vi "prediction_puissance.vi"() -> ()   [LabVIEW 2019]
uses:
  <vilib>/Utility/file.llb/Read Delimited Spreadsheet (DBL).vi
  <vilib>/Analysis/NI_AALPro.lvlib
panel:
  in  "Dossier ratio longueur d'ondes":path
  out "longueur d'onde":dbl
  out "XY Graph":cluster{"Y":dbl[], "Y":dbl[]}[](graph)
  in  "Dossier de tension":path
  # "on peut le remplacer par une constante dans le code"
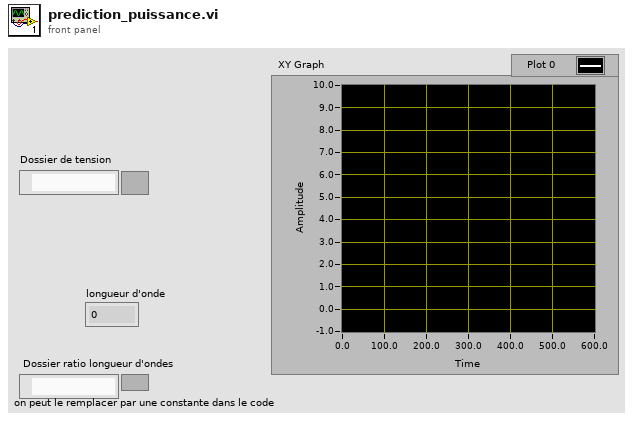
[diagram p1: front panel]
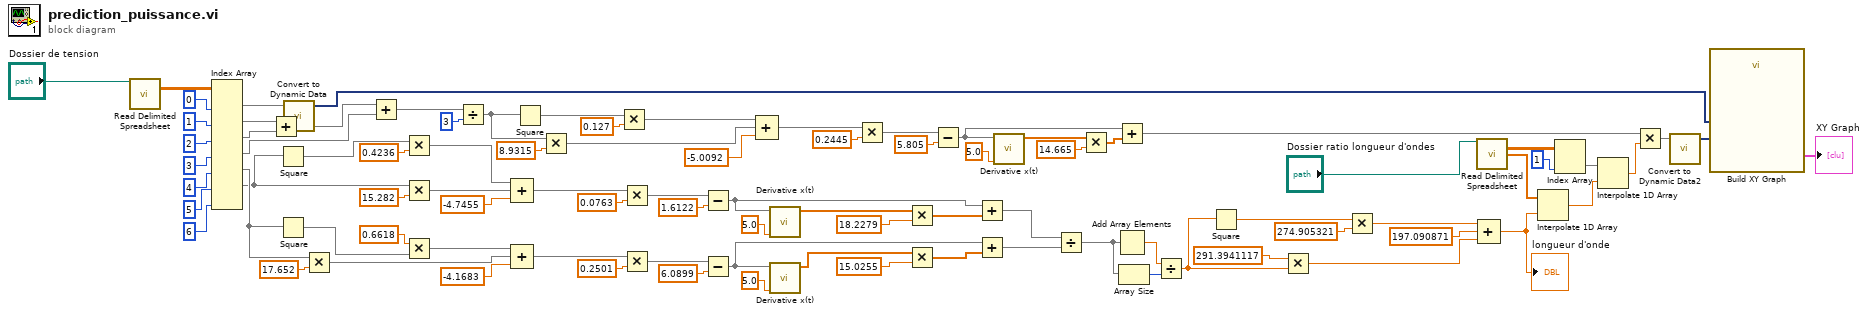
[diagram p0: block diagram]
diagram:
  n1 = call-poly <vilib>:"Read Delimited Spreadsheet.vi"("file path (dialog if empty)"="Dossier de tension") -> ("all rows"=w88:dbl[][])  [unwired: 9 in, 5 out]
  n2 = Index Array(array=w88, index (col) #1=0 ("disabled index (col)"), index (col) #2=1 ("index (col)"), index (col) #3=2 ("index (col)"), index (col) #4=3 ("index (col)"), index (col) #5=4 ("index (col)"), index (col) #6=5 ("index (col)"), index (col) #7=6 ("index (col)")) -> (element #1=w3:dbl[], element #2=w80:dbl[], element #3=w68:dbl[], element #4=w67:dbl[], element #5=w16:dbl[], element #6=w7:dbl[])  [unwired: 7 in, 1 out]
  n3 = Add(x=w80, y=w68) -> (x+y=w78:dbl[])
  n4 = Square(x=w7) -> (x^2=w6:dbl[])
  n5 = Square(x=w16) -> (x^2=w19:dbl[])
  n6 = call "Convert to Dynamic Data"("Array"=w3) -> ("Dynamic Data Type"=w49:dynamicdata)  [unwired: 3 in]
  n7 = Multiply(x=w16, y=17.652) -> (x*y=w14:dbl[])
  n8 = Add(x=w78, y=w67) -> (x+y=w79:dbl[])
  n9 = Multiply(x=w6, y=0.4236) -> (x*y=w5:dbl[])
  n10 = Multiply(x=w7, y=15.282) -> (x*y=w8:dbl[])
  n11 = Multiply(x=0.6618, y=w19) -> (x*y=w17:dbl[])
  n12 = Divide(x=w79, y=3) -> (x/y=w23:dbl[])
  n13 = Compound Arithmetic op=ADD(w5, w8, -4.7455) -> (w11:dbl[])
  n14 = Compound Arithmetic op=ADD(w17, w14, -4.1683) -> (w12:dbl[])
  n15 = Square(x=w23) -> (x^2=w26:dbl[])
  n16 = Multiply(x=w23, y=8.9315) -> (x*y=w21:dbl[])
  n17 = Multiply(x=w26, y=0.127) -> (x*y=w24:dbl[])
  n18 = Multiply(x=w11, y=0.0763) -> (x*y=w57:dbl[])
  n19 = Multiply(x=w12, y=0.2501) -> (x*y=w65:dbl[])
  n20 = Subtract(x=w57, y=1.6122) -> (x-y=w52:dbl[])
  n21 = Subtract(x=w65, y=6.0899) -> (x-y=w60:dbl[])
  n22 = Compound Arithmetic op=ADD(w24, w21, -5.0092) -> (w2:dbl[])
  n23 = call <vilib>:"Derivative x(t).vi"("dt"=5.0, "X"=w52) -> ("dX/dt"=w54:dbl[])  [unwired: 8 in, 1 out]
  n24 = call <vilib>:"Derivative x(t).vi"("dt"=5.0, "X"=w60) -> ("dX/dt"=w62:dbl[])  [unwired: 8 in, 1 out]
  n25 = Multiply(x=w2, y=0.2445) -> (x*y=w75:dbl[])
  n26 = Multiply(x=w54, y=18.2279) -> (x*y=w51:dbl[])
  n27 = Multiply(x=w62, y=15.0255) -> (x*y=w59:dbl[])
  n28 = Subtract(x=w75, y=5.805) -> (x-y=w70:dbl[])
  n29 = Add(x=w52, y=w51) -> (x+y=w37:dbl[])
  n30 = Add(x=w60, y=w59) -> (x+y=w38:dbl[])
  n31 = call <vilib>:"Derivative x(t).vi"("dt"=5.0, "X"=w70) -> ("dX/dt"=w72:dbl[])  [unwired: 8 in, 1 out]
  n32 = Divide(x=w37, y=w38) -> (x/y=w39:dbl[])
  n33 = Multiply(x=w72, y=14.665) -> (x*y=w69:dbl[])
  n34 = Add(x=w70, y=w69) -> (x+y=w1:dbl[])
  n35 = Add Array Elements(numeric array=w39) -> (sum=w41:dbl)
  n36 = Array Size(array=w39) -> (size(s)=w40:i32)
  n37 = Divide(x=w41, y=w40) -> (x/y=w36:dbl)
  n38 = Square(x=w36) -> (x^2=w47:dbl)
  n39 = Multiply(x=291.3941117, y=w36) -> (x*y=w43:dbl)
  n40 = Multiply(x=w47, y=274.905321) -> (x*y=w44:dbl)
  n41 = call-poly <vilib>:"Read Delimited Spreadsheet.vi"("file path (dialog if empty)"="Dossier ratio longueur d'ondes") -> ("all rows"=w31:dbl[][], "first row"=w34:dbl[])  [unwired: 9 in, 4 out]
  n42 = Compound Arithmetic op=ADD(w44, 197.090871, w43) -> (w35:dbl)
  "longueur d'onde" <- w35
  n43 = Interpolate 1D Array(1:w35, 2:w34) -> (0:w32:dbl)
  n44 = Index Array(array=w31, index (col)=1) -> (element=w29:dbl[])  [unwired: 1 in]
  n45 = Interpolate 1D Array(1:w32, 2:w29) -> (0:w27:dbl)
  n46 = Multiply(x=w1, y=w27) -> (x*y=w28:dbl[])
  n47 = call "Convert to Dynamic Data2"("Array"=w28) -> ("Dynamic Data Type"=w48:dynamicdata)  [unwired: 3 in]
  n48 = call "Build XY Graph"("Y Input"=w48, "X Input"=w49) -> ("XY Graph"=→"XY Graph":cluster{"X":dbl[], "Y":dbl[]}[])  [unwired: 8 in, 1 out]
